vi "Math Algos 3.vi"(9 "Measurements 2":T1, 11 "W (from Top View Algo)":dbl[](array[numeric]) format="%#_13g") -> (3 "H corrected":dbl[](array[numeric]))   [LabVIEW 2019, in "Algorithm.lvclass"]
uses:
  FrameworkOverrides/Algorithm.lvclass
  Controls/Measurements JSON Read.ctl
panel:
  out "NumericAray":i32[][](array[numeric])
  out "MeasurementIndices":i32[][](array[numeric])
  out "Array":string[](array[string])
  out "Alpha":dbl[](array[numeric])
  out "Thickness":dbl[](array[numeric])
  out "CurlGap":dbl[](array[numeric])
  out "Radius":dbl[](array[numeric])
  out "CamID":i32[](array[numeric])=[0, 0, 0, 1, 2, 1, 2, 1, 2, 1, 2, 0, 1, 2, 1, 2]
  out "Htrig":dbl[](array[numeric])
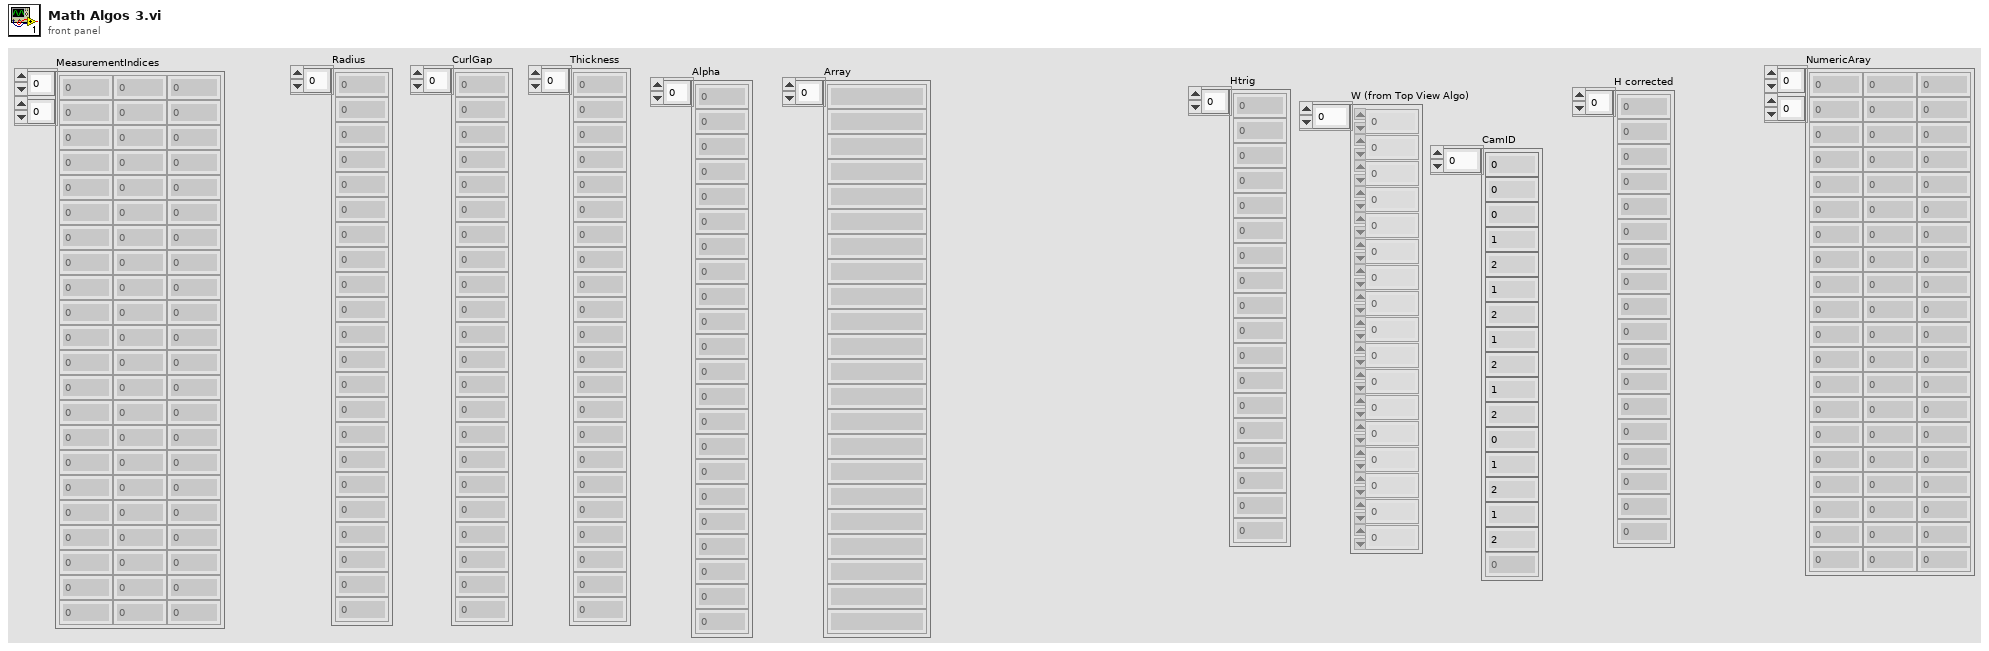
[diagram p1: front panel]
types:
  T1 = typedef "Algorithm.lvclass/Measurements JSON Read.ctl" = cluster{"RackID":i32, "ImageID":i32, "CameraID":i32, "MeasurementId":i32, "Name":string, "AlgoName":string, "Type":string, "MeasurementEnable":bool, "AlgorithmSequence":cluster{"RefernceEdge":cluster{"Enable":bool, "Method":string, "RefROI":cluster{"Left":i32, "Top":i32, "Right":i32, "Bottom":i32, "Rotation":dbl}, "EdgeOptions":cluster{"EdgePoarity":i32, "KernelSize":i32, "Width":i32, "MinimumEdgeStrength":i32, "InterpolationType":i32, "DataProcessingMethod":i32}, "LineOptions":cluster{"NumberofLines":i32, "Type":i32, "MinScore":i32, "MaxScore":i32, "Orientation":i32, "AngleRange":i32, "AngleTolerance":i32, "StepSize":i32, "MinSNR":i32, "MinPoints":i32, "HoughIterations":i32}, "SearchDirection":i32}, "Measurement":cluster{"ROI1":cluster{"Enable":bool, "ROI":cluster{"Left":i32, "Top":i32, "Right":i32, "Bottom":i32, "Rotation":dbl}, "EdgeOptions":cluster{"EdgePoarity":i32, "KernelSize":i32, "Width":i32, "MinimumEdgeStrength":i32, "InterpolationType":i32, "DataProcessingMethod":i32}, "LineOptions":cluster{"NumberofLines":i32, "Type":i32, "MinScore":i32, "MaxScore":i32, "Orientation":i32, "AngleRange":i32, "AngleTolerance":i32, "StepSize":i32, "MinSNR":i32, "MinPoints":i32, "HoughIterations":i32}, "Process":i32, "StepSize":i32, "SearchDirection":i32, "CircleEdgeOptions":cluster{"SearchDirection":i32, "EdgeOptions":cluster{"EdgePoarity":i32, "KernelSize":i32, "Width":i32, "MinimumEdgeStrength":i32, "InterpolationType":i32, "DataProcessingMethod":i32}}, "CircleFitOptions":cluster{"Process":i32, "StepSize":i32, "MAxPixelRadius":dbl}, "CircleSearchDirection":i32, "CurveParameters":cluster{"ExtractionMode":i32, "EdgeThreshold":i32, "EdgeFilterSize":i32, "MinLength":i32, "RowSearchStepSize":i32, "ColSearchStepSize":i32, "MaxEndpointGap":i32, "Closed":bool, "Subpixel":bool}, "MinimumMatchScore":i32, "CircleDescriptor":cluster{"MinRadius":i32, "MaxRadius":i32}, "EllipseDescriptor":cluster{"MinMajorRadius":i32, "MaxMajorRadius":i32, "MinMinorRadius":i32, "MaxMinorRadius":i32}}, "ROI2":cluster{"Enable":bool, "ROI":cluster{"Left":i32, "Top":i32, "Right":i32, "Bottom":i32, "Rotation":dbl}, "EdgeOptions":cluster{"EdgePoarity":i32, "KernelSize":i32, "Width":i32, "MinimumEdgeStrength":i32, "InterpolationType":i32, "DataProcessingMethod":i32}, "LineOptions":cluster{"NumberofLines":i32, "Type":i32, "MinScore":i32, "MaxScore":i32, "Orientation":i32, "AngleRange":i32, "AngleTolerance":i32, "StepSize":i32, "MinSNR":i32, "MinPoints":i32, "HoughIterations":i32}, "Process":i32, "StepSize":i32, "SearchDirection":i32, "CircleEdgeOptions":cluster{"SearchDirection":i32, "EdgeOptions":cluster{"EdgePoarity":i32, "KernelSize":i32, "Width":i32, "MinimumEdgeStrength":i32, "InterpolationType":i32, "DataProcessingMethod":i32}}, "CircleFitOptions":cluster{"Process":i32, "StepSize":i32, "MAxPixelRadius":dbl}, "CircleSearchDirection":i32, "CurveParameters":cluster{"ExtractionMode":i32, "EdgeThreshold":i32, "EdgeFilterSize":i32, "MinLength":i32, "RowSearchStepSize":i32, "ColSearchStepSize":i32, "MaxEndpointGap":i32, "Closed":bool, "Subpixel":bool}, "MinimumMatchScore":i32, "CircleDescriptor":cluster{"MinRadius":i32, "MaxRadius":i32}, "EllipseDescriptor":cluster{"MinMajorRadius":i32, "MaxMajorRadius":i32, "MinMinorRadius":i32, "MaxMinorRadius":i32}}}}, "MathExpression":cluster{"Algorithm":string, "MathExpression":string, "ResultVariable":string}, "MathCorrectionParameters":cluster{"Radius":dbl, "CurlGap":dbl, "Thickness":dbl, "MeasurementIndices":i32[], "MathAlgoName":string, "MathAlgoFormula":string, "CorrectionForAngle":i32[], "NumericAray":i32[], "StringArray":string[]}, "ResultVariableCluster":cluster{"RVName":string, "RVSequence":string, "RVIndex":i32, "RVID":i32, "RVValue":dbl}, "CalibrationCoefficients":cluster{"A1":dbl, "A2":dbl, "A3":dbl}, "UserCalibCoefficients":cluster{"UserCorrectionLinearityCoeff":dbl, "UserCorrectionBiasCoeff":dbl}, "SpecValues":cluster{"LCL":dbl, "UCL":dbl, "LSL":dbl, "USL":dbl, "NominalValue":dbl}, "OverlayOptions":cluster{"OverlayEnable":bool, "OverlayText":string, "OverlayCoords":i32[], "OverlayAngle":i32, "OverlayTextSize":i32, "OverlayTextColor":string, "OverlayROI":bool, "OverlayRakeLine":bool, "OverlayPoints":bool}, "DatalogEnable":bool, "DisplayIcon":string}[]
  T2 = cluster{"Radius":dbl, "CurlGap":dbl, "Thickness":dbl, "MeasurementIndices":i32[], "MathAlgoName":string, "MathAlgoFormula":string, "CorrectionForAngle":i32[], "NumericAray":i32[], "StringArray":string[]}
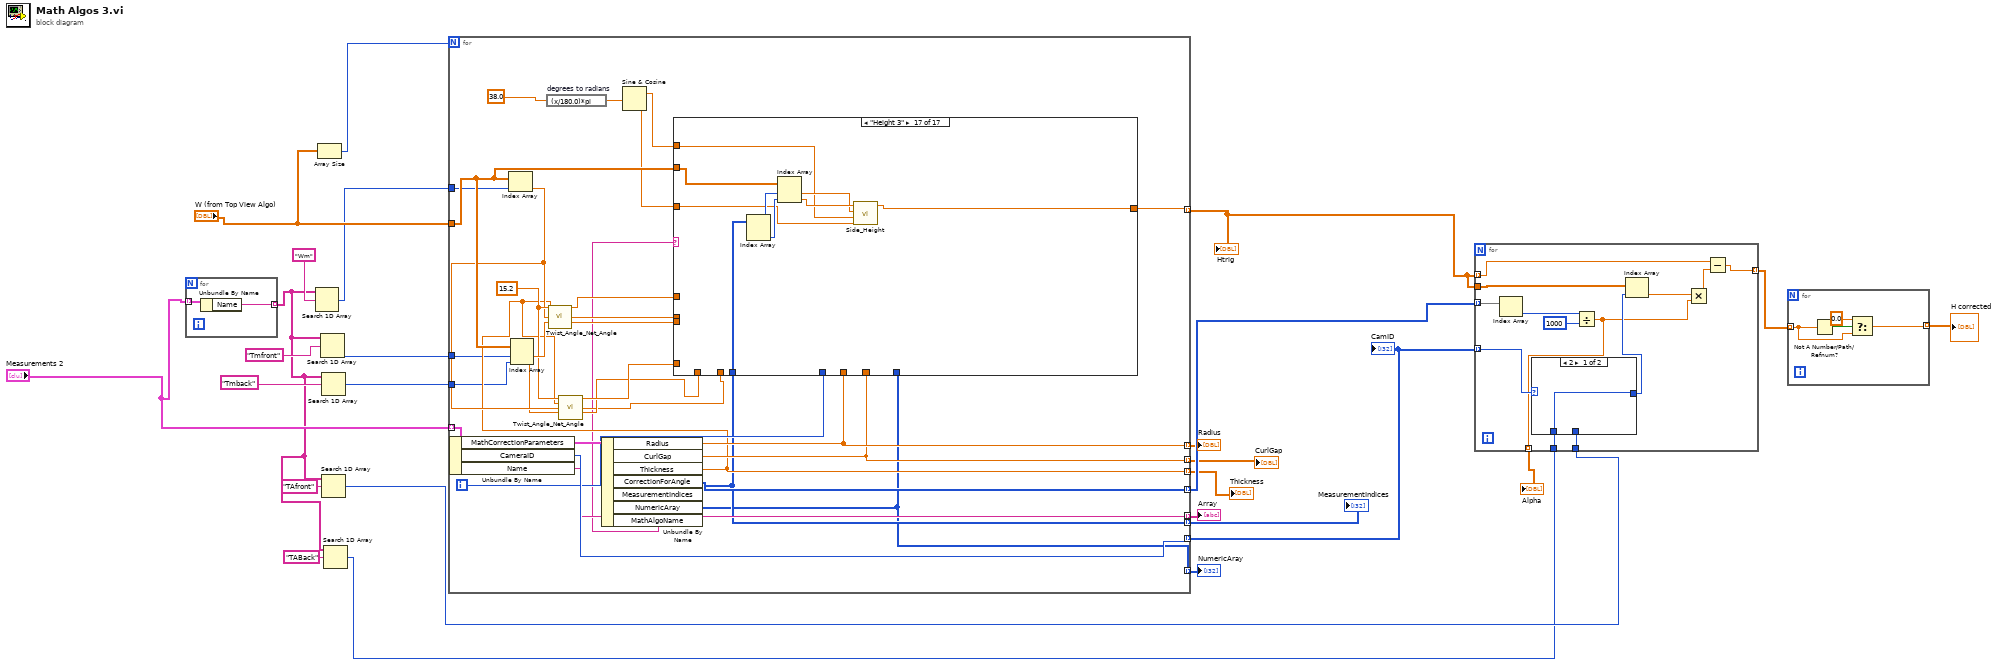
[diagram p0: block diagram]
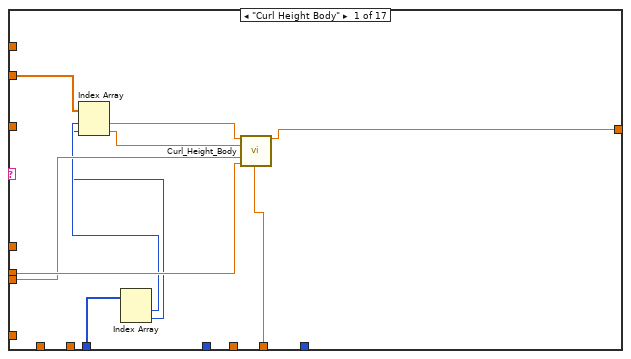
[diagram p3: hidden frame]
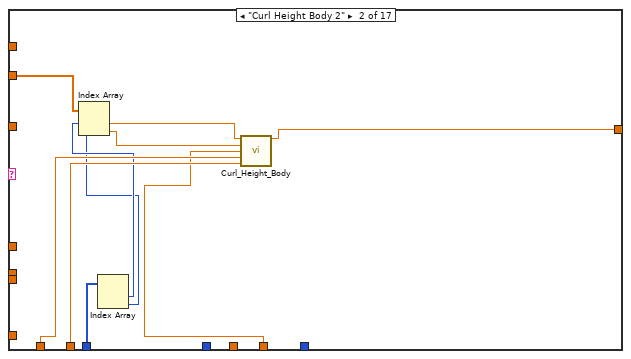
[diagram p4: hidden frame]
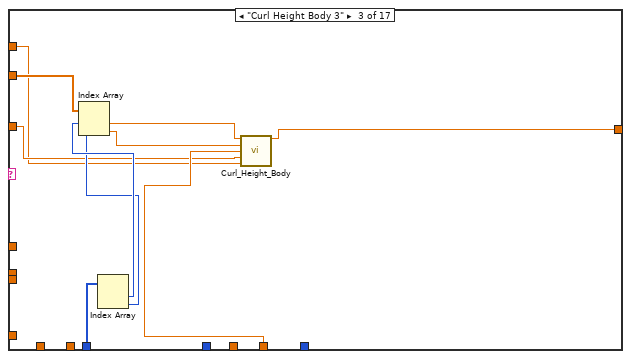
[diagram p5: hidden frame]
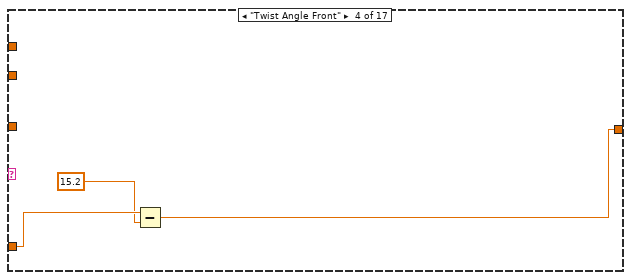
[diagram p6: hidden frame]
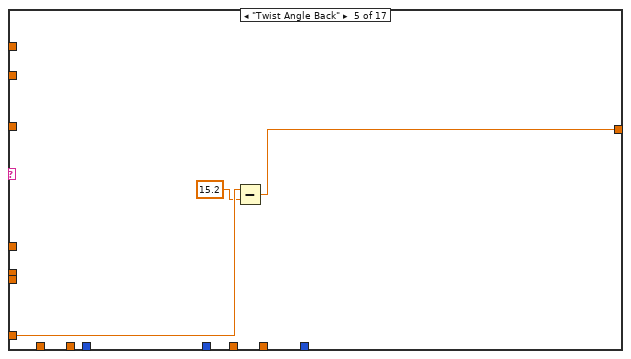
[diagram p7: hidden frame]
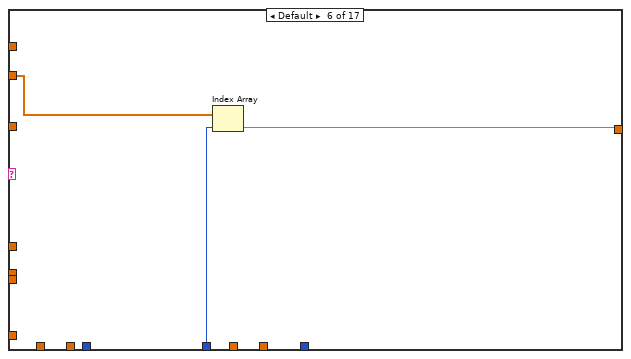
[diagram p8: hidden frame]
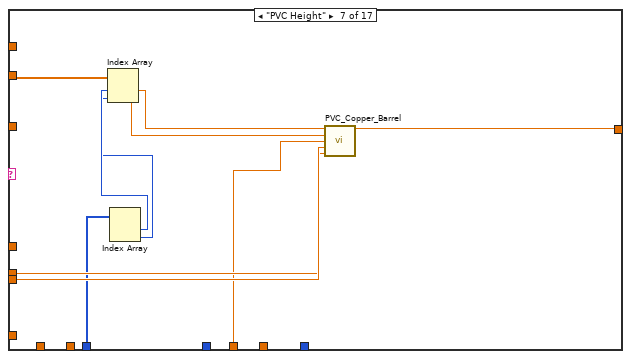
[diagram p9: hidden frame]
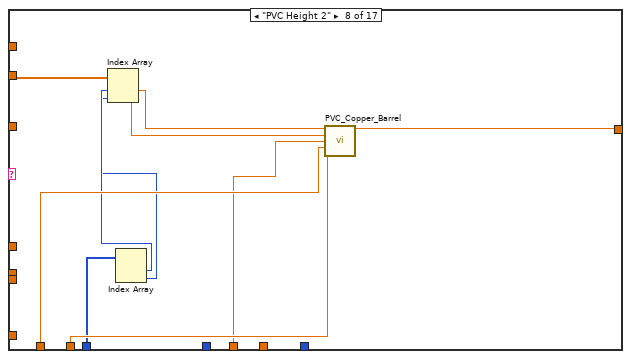
[diagram p10: hidden frame]
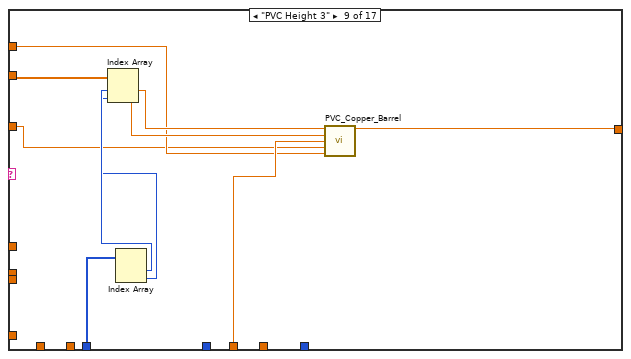
[diagram p11: hidden frame]
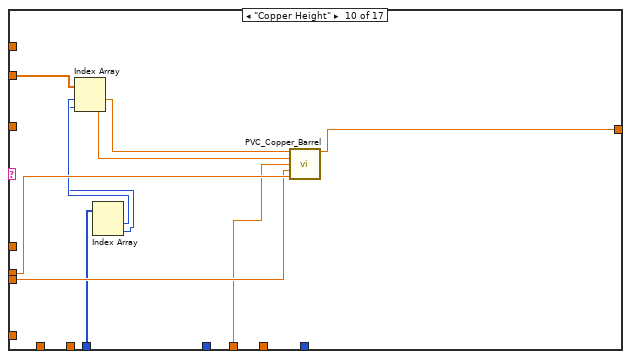
[diagram p12: hidden frame]
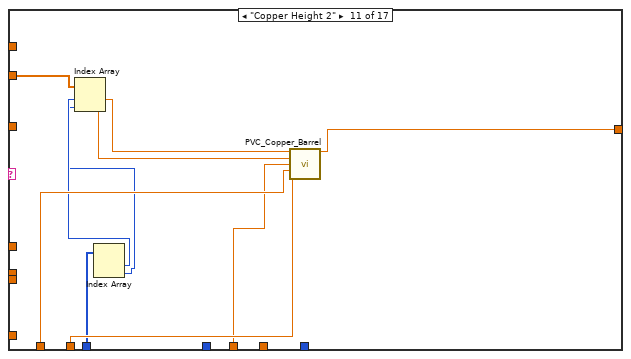
[diagram p13: hidden frame]
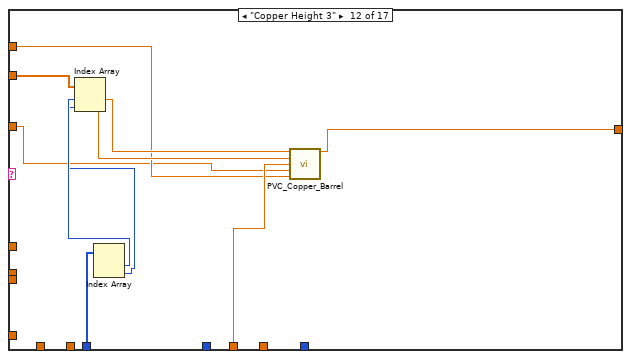
[diagram p14: hidden frame]
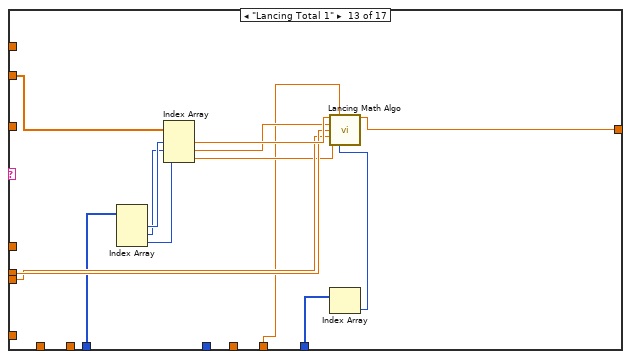
[diagram p15: hidden frame]
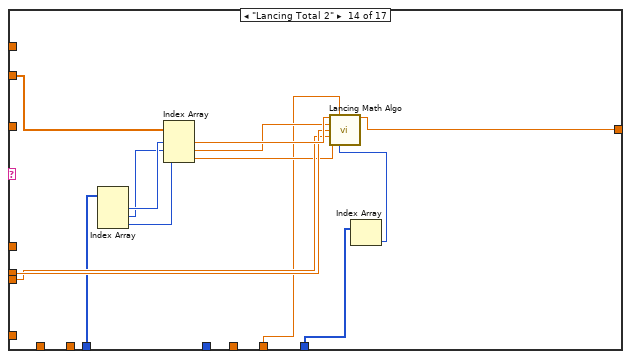
[diagram p16: hidden frame]
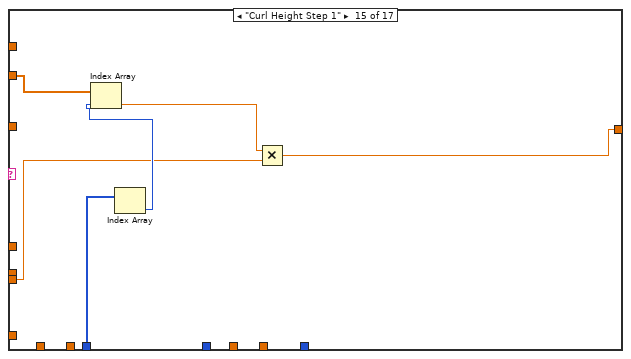
[diagram p17: hidden frame]
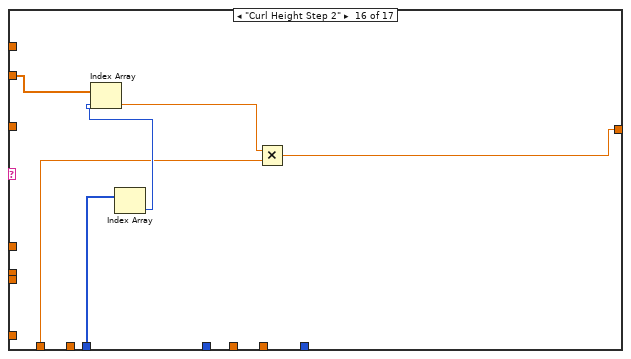
[diagram p18: hidden frame]
diagram:
  n1 = for {
    tunnel: "Measurements 2" -> [w28] mode=indexing
    tunnel: [w27] -> w5 mode=indexing
    n2 = Unbundle By Name(w28) -> ("Name"=w27:string)
  }
  n3 = Search 1D Array(1D array=w5, element="Wm") -> (index of element=w11:i32)  [unwired: 1 in]
  n4 = Array Size(array="W (from Top View Algo)") -> (size(s)=w26:i32)
  n5 = Search 1D Array(1D array=w5, element="Tmfront") -> (index of element=w9:i32)  [unwired: 1 in]
  n6 = Search 1D Array(1D array=w5, element="Tmback") -> (index of element=w7:i32)  [unwired: 1 in]
  n7 = Search 1D Array(1D array=w5, element="TAfront") -> (index of element=w3:i32)  [unwired: 1 in]
  n8 = Search 1D Array(1D array=w5, element="TABack") -> (index of element=w2:i32)  [unwired: 1 in]
  n9 = for {
    N: w26 -> [_]
    tunnel: "W (from Top View Algo)" -> [w59]
    tunnel: [w56] -> w24 mode=indexing
    tunnel: "Measurements 2" -> [w47] mode=indexing
    tunnel: [w45] -> w21 mode=indexing
    tunnel: [w44] -> w20 mode=indexing
    tunnel: [w42] -> w19 mode=indexing
    tunnel: [w41] -> w18 mode=indexing
    tunnel: [w40] -> w17 mode=indexing
    tunnel: [w39] -> w15 mode=indexing
    tunnel: [w38] -> w14 mode=indexing
    tunnel: w11 -> [w37]
    tunnel: w9 -> [w36]
    tunnel: w7 -> [w35]
    tunnel: [w34] -> w1 mode=indexing
    i -> [w43]
    w50 = 15.2 ("Theta_c")
    n10 = Unbundle By Name(w47) -> ("MathCorrectionParameters"=w46:T2, "CameraID"=w45:i32, "Name"=w39:string)
    n11 = Index Array(array=w59, index=w37) -> (element=w49:dbl)
    n12 = Index Array(array=w59, index #1=w36, index #2=w35) -> (element #1=w54:dbl, element #2=w48:dbl)
    n13 = expression code="(x/180.0)*pi" "degrees to radians"(38.0 ("Theta_c")) -> (w32:dbl)
    n14 = Unbundle By Name(w46) -> ("Radius"=w42:dbl, "CurlGap"=w41:dbl, "Thickness"=w40:dbl, "CorrectionForAngle"=w44:i32[], "MeasurementIndices"=w38:i32[], "NumericAray"=w34:i32[], "MathAlgoName"=w29:string)
    n15 = call "Twist_Angle_Net_Angle.vi"("Theta_c"=w50, "Neck Thickness"=w40, "Wm"=w49, "Tm"=w54) -> ("Net"=w55:dbl, "Sine_Net"=w58:dbl, "Cosine_Net"=w57:dbl)  [unwired: 8 in, 1 out]
    n16 = call "Twist_Angle_Net_Angle.vi"("Theta_c"=w50, "Neck Thickness"=w40, "Wm"=w49, "Tm"=w48) -> ("Net"=w53:dbl, "Sine_Net"=w51:dbl, "Cosine_Net"=w52:dbl)  [unwired: 8 in, 1 out]
    n17 = Sine & Cosine(0:w32) -> (1:w31:dbl, 2:w30:dbl)
    n18 = case shown="\"Height 3\"" w29 {
      tunnel: w59 -> [w69 w79 w89 _ _ w97 w107 w117 w127 w137 w147 w157 w172 w186 w192 w198 w207]
      tunnel: w58 -> [w66 _ _ _ _ _ w103 _ _ w134 _ _ w169 w183 _ _ _]
      tunnel: w57 -> [w65 _ _ _ _ _ w104 _ _ w133 _ _ w168 w182 w187 _ _]
      tunnel: [w64 w76 w86 w92 w95 w96 w108 w118 w128 w138 w148 w158 w166 w180 w188 w194 w204] -> w56
      tunnel: w43 -> [_ _ _ _ _ w98 _ _ _ _ _ _ _ _ _ _ _]
      tunnel: w55 -> [_ _ _ w91 _ _ _ _ _ _ _ _ _ _ _ _ _]
      tunnel: w53 -> [_ _ _ _ w94 _ _ _ _ _ _ _ _ _ _ _ _]
      tunnel: w52 -> [_ w74 _ _ _ _ _ w114 _ _ w144 _ _ _ _ w193 _]
      tunnel: w51 -> [_ w75 _ _ _ _ _ w113 _ _ w143 _ _ _ _ _ _]
      tunnel: w42 -> [_ _ _ _ _ _ w102 w112 w124 w132 w142 w154 _ _ _ _ _]
      tunnel: w41 -> [w63 w73 w85 _ _ _ _ _ _ _ _ _ w165 w179 _ _ _]
      tunnel: w38 -> [w62 w72 w84 _ _ _ w101 w111 w123 w131 w141 w153 w164 w178 w191 w197 w206]
      tunnel: w34 -> [_ _ _ _ _ _ _ _ _ _ _ _ w160 w174 _ _ _]
      tunnel: w31 -> [_ _ w80 _ _ _ _ _ w120 _ _ w150 _ _ _ _ w200]
      tunnel: w30 -> [_ _ w81 _ _ _ _ _ w119 _ _ w149 _ _ _ _ w199]
      frame "Curl Height Body" {
        n19 = Index Array(array=w62) -> (element #1=w61:i32, element #2=w60:i32)  [unwired: 2 in]
        n20 = Index Array(array=w69, index #1=w61, index #2=w60) -> (element #1=w68:dbl, element #2=w67:dbl)
        n21 = call "Curl_Height_Body.vi"("Wm"=w68, "Hm"=w67, "Curl Gap"=w63, "cos_net"=w65, "sin_net"=w66) -> ("H"=w64:dbl)  [unwired: 10 in]
      }
      frame "Curl Height Body 2" {
        n22 = Index Array(array=w72) -> (element #1=w71:i32, element #2=w70:i32)  [unwired: 2 in]
        n23 = Index Array(array=w79, index #1=w71, index #2=w70) -> (element #1=w78:dbl, element #2=w77:dbl)
        n24 = call "Curl_Height_Body.vi"("Wm"=w78, "Hm"=w77, "Curl Gap"=w73, "cos_net"=w74, "sin_net"=w75) -> ("H"=w76:dbl)  [unwired: 10 in]
      }
      frame "Curl Height Body 3" {
        n25 = Index Array(array=w84) -> (element #1=w83:i32, element #2=w82:i32)  [unwired: 2 in]
        n26 = Index Array(array=w89, index #1=w83, index #2=w82) -> (element #1=w88:dbl, element #2=w87:dbl)
        n27 = call "Curl_Height_Body.vi"("Wm"=w88, "Hm"=w87, "Curl Gap"=w85, "cos_net"=w81, "sin_net"=w80) -> ("H"=w86:dbl)  [unwired: 10 in]
      }
      frame "Twist Angle Front" {
        n28 = Subtract(x=w91, y=15.2) -> (x-y=w92:dbl)
      }
      frame "Twist Angle Back" {
        n29 = Subtract(x=w94, y=15.2 ("x")) -> (x-y=w95:dbl)
      }
      frame Default {
        n30 = Index Array(array=w97, index=w98) -> (element=w96:dbl)
      }
      frame "PVC Height" {
        n31 = Index Array(array=w101) -> (element #1=w100:i32, element #2=w99:i32)  [unwired: 2 in]
        n32 = Index Array(array=w107, index #1=w100, index #2=w99) -> (element #1=w106:dbl, element #2=w105:dbl)
        n33 = call "PVC_Copper_Barrel.vi"("Wm"=w106, "Hm"=w105, "R"=w102, "Cos_net"=w104, "Sin_net"=w103) -> ("height"=w108:dbl)  [unwired: 10 in]
      }
      frame "PVC Height 2" {
        n34 = Index Array(array=w111) -> (element #1=w110:i32, element #2=w109:i32)  [unwired: 2 in]
        n35 = Index Array(array=w117, index #1=w110, index #2=w109) -> (element #1=w116:dbl, element #2=w115:dbl)
        n36 = call "PVC_Copper_Barrel.vi"("Wm"=w116, "Hm"=w115, "R"=w112, "Cos_net"=w114, "Sin_net"=w113) -> ("height"=w118:dbl)  [unwired: 10 in]
      }
      frame "PVC Height 3" {
        n37 = Index Array(array=w123) -> (element #1=w122:i32, element #2=w121:i32)  [unwired: 2 in]
        n38 = Index Array(array=w127, index #1=w122, index #2=w121) -> (element #1=w126:dbl, element #2=w125:dbl)
        n39 = call "PVC_Copper_Barrel.vi"("Wm"=w126, "Hm"=w125, "R"=w124, "Cos_net"=w119, "Sin_net"=w120) -> ("height"=w128:dbl)  [unwired: 10 in]
      }
      frame "Copper Height" {
        n40 = Index Array(array=w131) -> (element #1=w130:i32, element #2=w129:i32)  [unwired: 2 in]
        n41 = Index Array(array=w137, index #1=w130, index #2=w129) -> (element #1=w136:dbl, element #2=w135:dbl)
        n42 = call "PVC_Copper_Barrel.vi"("Wm"=w136, "Hm"=w135, "R"=w132, "Cos_net"=w133, "Sin_net"=w134) -> ("height"=w138:dbl)  [unwired: 10 in]
      }
      frame "Copper Height 2" {
        n43 = Index Array(array=w141) -> (element #1=w140:i32, element #2=w139:i32)  [unwired: 2 in]
        n44 = Index Array(array=w147, index #1=w140, index #2=w139) -> (element #1=w146:dbl, element #2=w145:dbl)
        n45 = call "PVC_Copper_Barrel.vi"("Wm"=w146, "Hm"=w145, "R"=w142, "Cos_net"=w144, "Sin_net"=w143) -> ("height"=w148:dbl)  [unwired: 10 in]
      }
      frame "Copper Height 3" {
        n46 = Index Array(array=w153) -> (element #1=w152:i32, element #2=w151:i32)  [unwired: 2 in]
        n47 = Index Array(array=w157, index #1=w152, index #2=w151) -> (element #1=w156:dbl, element #2=w155:dbl)
        n48 = call "PVC_Copper_Barrel.vi"("Wm"=w156, "Hm"=w155, "R"=w154, "Cos_net"=w149, "Sin_net"=w150) -> ("height"=w158:dbl)  [unwired: 10 in]
      }
      frame "Lancing Total 1" {
        n49 = Index Array(array=w164) -> (element #1=w163:i32, element #2=w162:i32, element #3=w161:i32)  [unwired: 3 in]
        n50 = Index Array(array=w172, index #1=w163, index #2=w162, index #3=w161) -> (element #1=w171:dbl, element #2=w170:dbl, element #3=w167:dbl)
        n51 = Index Array(array=w160) -> (element=w159:i32)  [unwired: 1 in]
        n52 = call "Lancing Math Algo.vi"("Wm"=w171, "Curl Gap"=w165, "Hm"=w170, "sin_net"=w169, "cos_net"=w168, "Hm'"=w167, "Lock Width"=w159) -> ("Lancing"=w166:dbl)  [unwired: 8 in]
      }
      frame "Lancing Total 2" {
        n53 = Index Array(array=w178) -> (element #1=w177:i32, element #2=w176:i32, element #3=w175:i32)  [unwired: 3 in]
        n54 = Index Array(array=w186, index #1=w177, index #2=w176, index #3=w175) -> (element #1=w185:dbl, element #2=w184:dbl, element #3=w181:dbl)
        n55 = Index Array(array=w174) -> (element=w173:i32)  [unwired: 1 in]
        n56 = call "Lancing Math Algo.vi"("Wm"=w185, "Curl Gap"=w179, "Hm"=w184, "sin_net"=w183, "cos_net"=w182, "Hm'"=w181, "Lock Width"=w173) -> ("Lancing"=w180:dbl)  [unwired: 8 in]
      }
      frame "Curl Height Step 1" {
        n57 = Index Array(array=w191) -> (element=w190:i32)  [unwired: 1 in]
        n58 = Index Array(array=w192, index=w190) -> (element=w189:dbl)
        n59 = Multiply(x=w189, y=w187) -> (x*y=w188:dbl)
      }
      frame "Curl Height Step 2" {
        n60 = Index Array(array=w197) -> (element=w196:i32)  [unwired: 1 in]
        n61 = Index Array(array=w198, index=w196) -> (element=w195:dbl)
        n62 = Multiply(x=w195, y=w193) -> (x*y=w194:dbl)
      }
      frame "Height 3" {
        n63 = Index Array(array=w206) -> (element #1=w205:i32, element #2=w203:i32)  [unwired: 2 in]
        n64 = Index Array(array=w207, index #1=w205, index #2=w203) -> (element #1=w201:dbl, element #2=w202:dbl)
        n65 = call "Side_Height.vi"("cos_theta"=w199, "sin_theta"=w200, "W"=w201, "H'"=w202) -> ("H"=w204:dbl)  [unwired: 7 in]
      }
    }
  }
  "Htrig" <- w24
  "CamID" <- w21
  "Radius" <- w19
  "CurlGap" <- w18
  "Thickness" <- w17
  "Array" <- w15
  "MeasurementIndices" <- w14
  "NumericAray" <- w1
  n66 = for {
    tunnel: w21 -> [w220] mode=indexing
    tunnel: w20 -> [w213] mode=indexing
    tunnel: w24 -> [w217] mode=indexing
    tunnel: w24 -> [w219]
    tunnel: [w214] -> w23 mode=indexing
    tunnel: [w210] -> w16 mode=indexing
    tunnel: w3 -> [w209]
    tunnel: w2 -> [w208]
    n67 = Index Array(array=w213) -> (element=w211:i32)  [unwired: 1 in]
    n68 = case shown="2" w220 {
      tunnel: [w221 w222] -> w218
      tunnel: w209 -> [_ w222]
      tunnel: w208 -> [w221 _]
      frame 2 {
      }
      frame 1, Default {
      }
    }
    n69 = Divide(x=w211, y=1000) -> (x/y=w210:dbl)
    n70 = Index Array(array=w219, index=w218) -> (element=w216:dbl)
    n71 = Multiply(x=w216, y=w210) -> (x*y=w215:dbl)
    n72 = Subtract(x=w217, y=w215) -> (x-y=w214:dbl)
  }
  "Alpha" <- w16
  n73 = for {
    tunnel: w23 -> [w225] mode=indexing
    tunnel: [w223] -> w22 mode=indexing
    n74 = Not A Number/Path/Refnum?(number/path/refnum=w225) -> (NaN/Path/Refnum?=w226:bool)
    n75 = Select(t=0.0, s=w226, f=w225) -> (s? t:f=w223:dbl)
  }
  "H corrected" <- w22
